vi "Turn90.vi"(8 "Right?":bool, 11 "Boolean in":bool) -> (3 "Boolean out":bool)   [LabVIEW 2014]
uses:
  Support Files/Global Data!!!.vi
  <vilib>/addons/control/pid/pid.llb/PID (DBL).vi
  <vilib>/addons/control/pid/NI_PID_pid.lvlib
panel:
  out "Boolean out 2":bool
  in  "Boolean in 2":bool
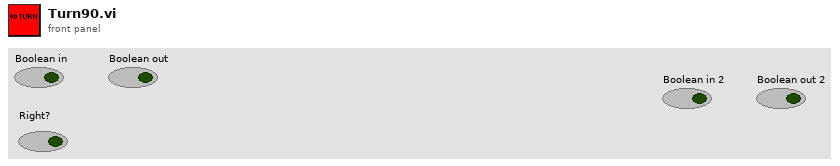
[diagram p1: front panel]
types:
  T1 = cluster{"proportional gain (Kc)":dbl, "integral time (Ti, min)":dbl, "derivative time (Td, min)":dbl}
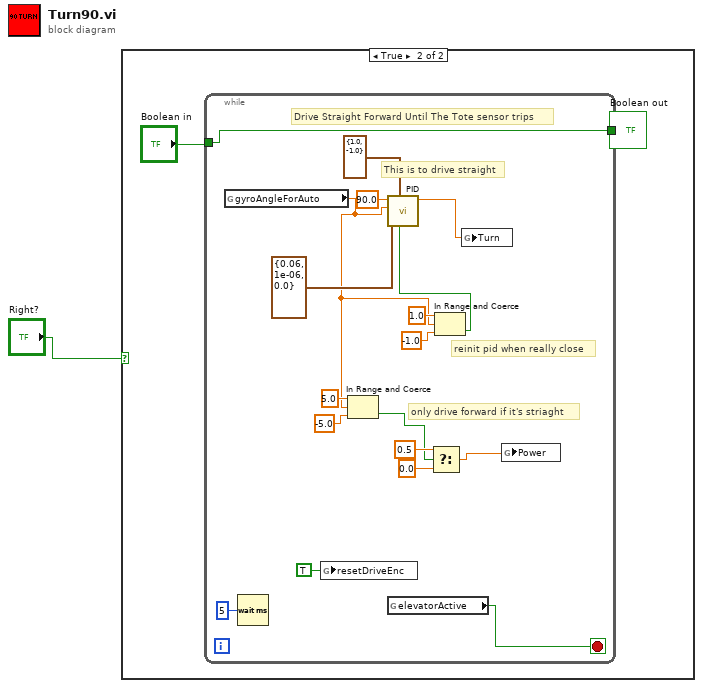
[diagram p0: block diagram]
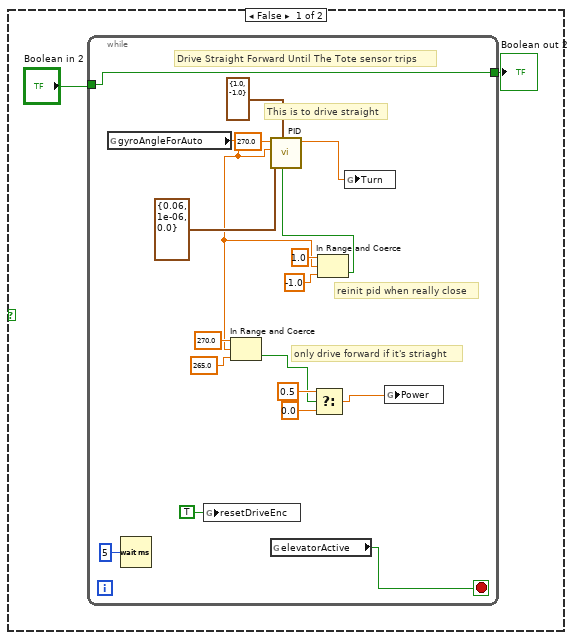
[diagram p2: hidden frame]
diagram:
  n1 = case shown="True" "Right?" {
    frame False {
      n2 = while {
        tunnel: [w5] -> w2
        tunnel: "Boolean in 2" -> [w5]
        stop <- w10 stop-if-true
        # "reinit pid when really close"
        # "Drive Straight Forward Until The Tote sensor trips"
        # "only drive forward if it's striaght"
        # "This is to drive straight"
        n3 = global read "Global Data!!!.vi" "gyroAngleForAuto"() -> (w7:dbl)
        n4 = Wait (ms)(milliseconds to wait=u32 5) -> ()  [unwired: 1 out]
        n5 = global write "Global Data!!!.vi" "resetDriveEnc"(TRUE ("resetDriveEnc")) -> ()
        n6 = In Range and Coerce(upper limit=270.0, x=w7, lower limit=265.0) -> (In Range?=w11:bool)  [unwired: 1 out]
        n7 = global read "Global Data!!!.vi" "elevatorActive"() -> (w10:bool)
        n8 = Select(t=0.5, s=w11, f=0.0) -> (s? t:f=w17:dbl)
        n9 = In Range and Coerce(upper limit=1.0, x=w7, lower limit=-1.0) -> (In Range?=w6:bool)  [unwired: 1 out]
        n10 = call-poly <vilib>:"PID.vi"("reinitialize? (F)"=w6, "output range"=cluster{"output high":dbl, "output low":dbl} {"output high"=1.0, "output low"=-1.0}, "PID gains"=T1 {"proportional gain (Kc)"=0.06, "integral time (Ti, min)"=1e-06, "derivative time (Td, min)"=0.0}, "process variable"=w7, "setpoint"=270.0) -> ("output"=w20:dbl)  [unwired: 5 in, 1 out]
        n11 = global write "Global Data!!!.vi" "Turn"(w20) -> ()
        n12 = global write "Global Data!!!.vi" "Power"(w17) -> ()
      }
      "Boolean out 2" <- w2
    }
    frame True {
      n13 = while {
        tunnel: [w25] -> w22
        tunnel: "Boolean in" -> [w25]
        stop <- w30 stop-if-true
        # "reinit pid when really close"
        # "Drive Straight Forward Until The Tote sensor trips"
        # "only drive forward if it's striaght"
        # "This is to drive straight"
        n14 = global read "Global Data!!!.vi" "gyroAngleForAuto"() -> (w27:dbl)
        n15 = Wait (ms)(milliseconds to wait=u32 5) -> ()  [unwired: 1 out]
        n16 = global write "Global Data!!!.vi" "resetDriveEnc"(TRUE ("resetDriveEnc")) -> ()
        n17 = In Range and Coerce(upper limit=5.0, x=w27, lower limit=-5.0) -> (In Range?=w31:bool)  [unwired: 1 out]
        n18 = global read "Global Data!!!.vi" "elevatorActive"() -> (w30:bool)
        n19 = Select(t=0.5, s=w31, f=0.0) -> (s? t:f=w37:dbl)
        n20 = In Range and Coerce(upper limit=1.0, x=w27, lower limit=-1.0) -> (In Range?=w26:bool)  [unwired: 1 out]
        n21 = call-poly <vilib>:"PID.vi"("reinitialize? (F)"=w26, "output range"=cluster{"output high":dbl, "output low":dbl} {"output high"=1.0, "output low"=-1.0}, "PID gains"=T1 {"proportional gain (Kc)"=0.06, "integral time (Ti, min)"=1e-06, "derivative time (Td, min)"=0.0}, "process variable"=w27, "setpoint"=90.0) -> ("output"=w40:dbl)  [unwired: 5 in, 1 out]
        n22 = global write "Global Data!!!.vi" "Turn"(w40) -> ()
        n23 = global write "Global Data!!!.vi" "Power"(w37) -> ()
      }
      "Boolean out" <- w22
    }
  }
